vi "ReCalc V0.09.vi"() -> ()   [LabVIEW 2014]
uses:
  <vilib>/Utility/miscctls.llb/LVPointTypeDef.ctl
  <vilib>/Utility/NIReport.llb/Append Report Text (str wrap).vi
  <vilib>/Utility/xml.llb/Write to XML File(string).vi
  <vilib>/Utility/xml.llb/Read From XML File(string).vi
  <vilib>/Analysis/3filter.llb/IIR Filter (DBL).vi
  <vilib>/Utility/NIReport.llb/NI_report.lvclass
  <vilib>/Analysis/NI_AALBase.lvlib
  <vilib>/Analysis/NI_AALPro.lvlib
panel:
  in  "Speichern":bool
  out "aus Getriebe & Reifen":bool
  out "aus Zündsignal":bool=TRUE
  out "Reifenumfang [m]":dbl=1.222
  out "Getriebe [1:]":dbl=5.343
  out "Zündung [Imp/U]":u8=1
  out "Rolle [Inkr/U]":u16=200
  out "Luftdruck [mbar]":dbl=1013.0
  out "Luftfeuchtigkeit [%]":dbl=50.0
  out "Lufttemperatur [°C]":dbl=20.0
  in  "Berechnen":bool
  in  "Stopp":bool
  in  "Rollenträgheit [kgm²]":dbl=0.402
  in  "Polynom":u8=15
  in  "Gl. Mittelwert":u8=35
  in  "Differenzenquotient":u8=12
  in  "n vom Gas [1/min]":dbl=5000.0
  out "Rollenumfang [m]":dbl=0.613 format="%.3f"
  in  "nmax [1/min]":dbl=11000.0
  in  "nmin [1/min]":dbl=3000.0
  out "Datum, Zeit":string
  out "Untersetzung:":dbl=2.68 format="%.2f"
  in  "Drucken":bool
  out "Pmax":string
  out "Ergebnis":string
  out "Fahrzeugdaten":string
  out "XY-Graph":cluster{dbl[], dbl[]}[](graph)
  in  "Öffnen":bool
  out "korr":dbl
  out "[s]":dbl=5.0
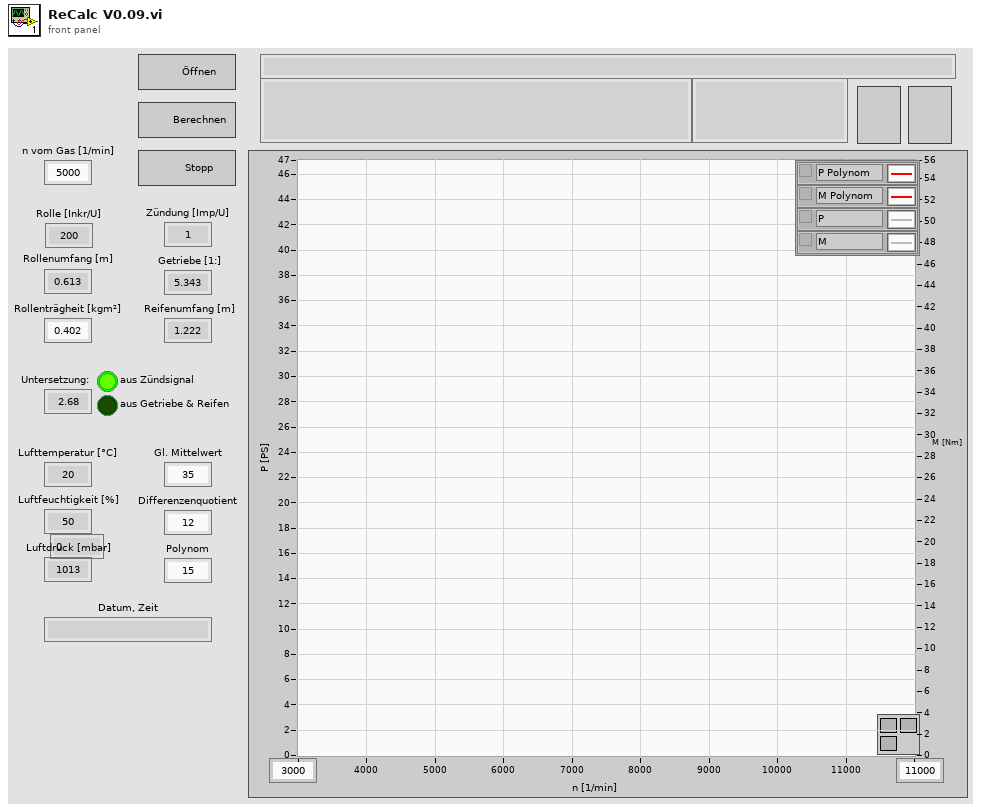
[diagram p1: front panel]
types:
  T1 = typedef "LVPointTypeDef.ctl" = cluster{"Horizontal":i16, "Vertical":i16}
  T2 = enum16{"Kleinste Quadrate", "Kleinestes absolutes Reiduum", "Biquadrat"}
  T3 = cluster{"Fahrzeugdaten":string, "Value":string, "Value":u16, "Value":dbl, "Value":dbl, "Value":u8, "Value":dbl, "Value":dbl, "Value":dbl, "Value":u8, "Value":u8, "Value":u8, dbl, dbl, "Value":dbl, "Value":dbl, "Value":dbl, dbl[], dbl[], "Best Polynomial Fit":dbl[], dbl[], "Value":bool, "Value":dbl, "Value":dbl, "Value":dbl, "Value":dbl, dbl[], i32[]}
  T4 = cluster{string, string, u16, dbl, dbl, u8, dbl, dbl, dbl, u8, u8, u8, dbl, dbl, dbl, dbl, dbl, dbl[], dbl[], dbl[], dbl[], bool, dbl, dbl, dbl, dbl, dbl[], i32[]}
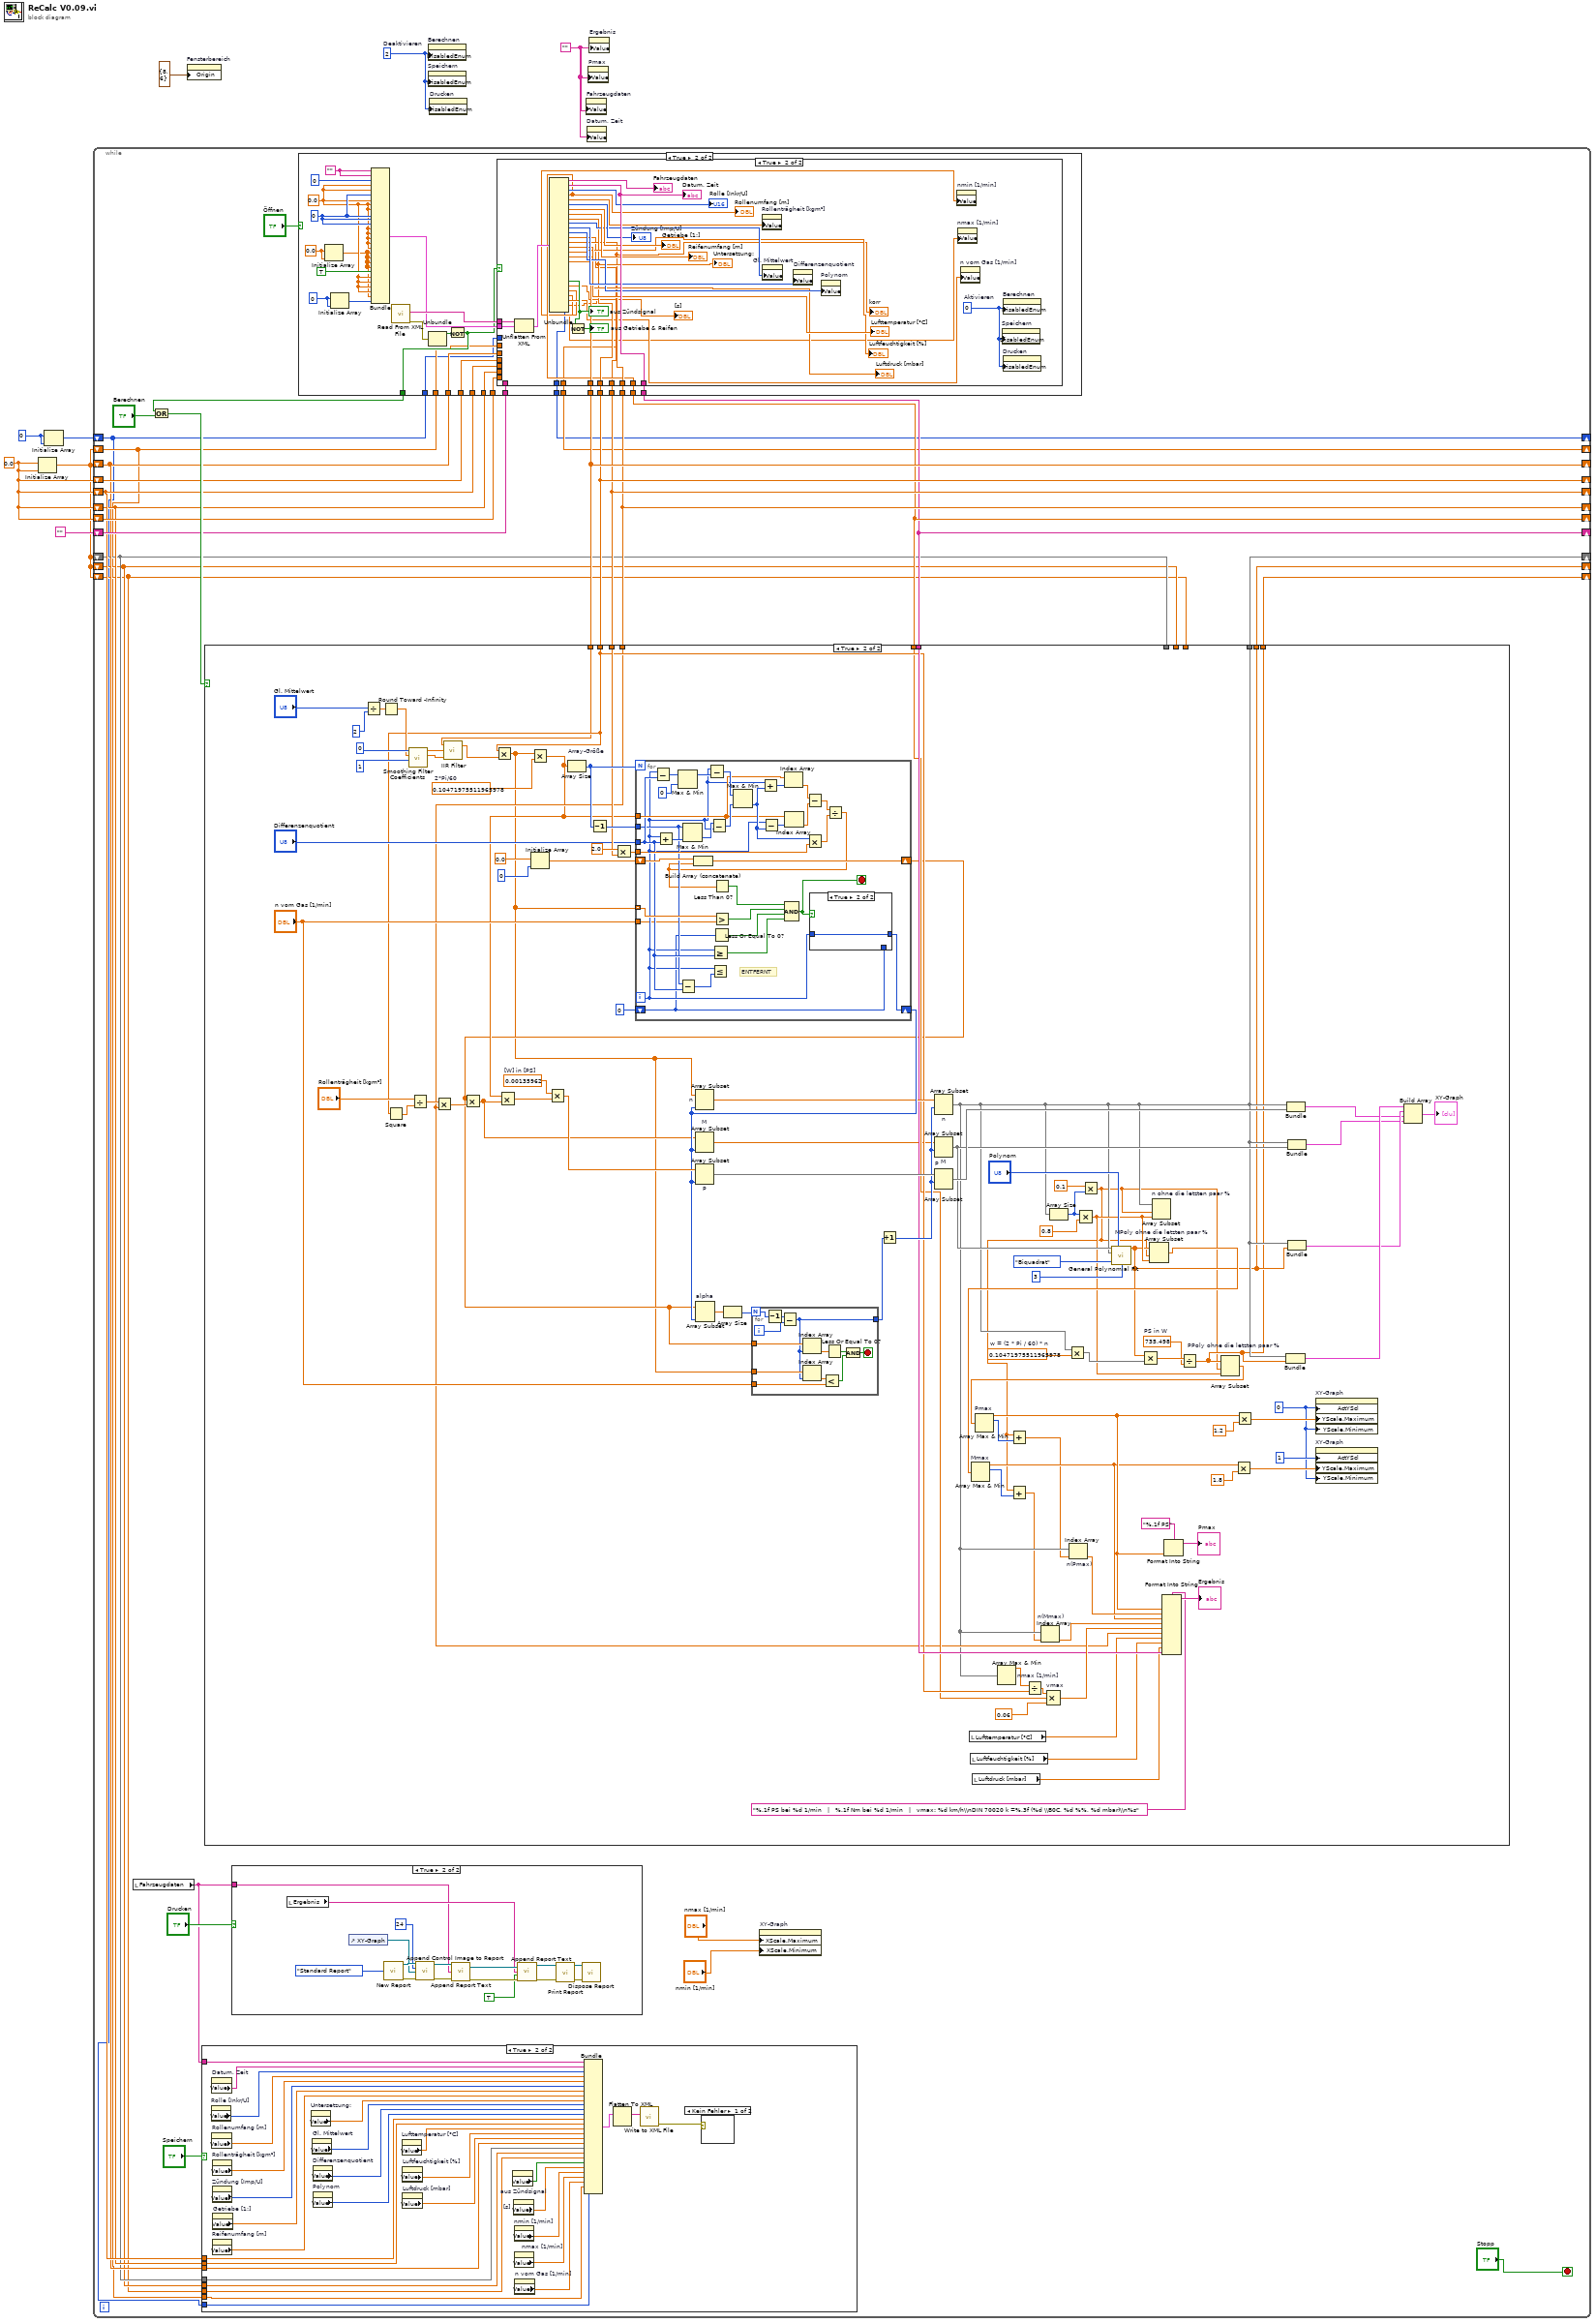
[diagram p0: block diagram]
diagram:
  w1 = 0
  w7 = 0.0
  w4 = 2  # Deaktivieren
  w8 = ""
  n1 = Initialize Array(w7, w7) -> (w3:dbl[])
  n2 = Initialize Array(w1, w1) -> (w2:i32[])
  n3 = while {
    shift-right: [w32] -> _
    shift-left: w3 -> [w21]
    shift-right: [w31] -> _
    shift-left: w7 -> [w35]
    shift-right: [w30] -> _
    shift-left: w7 -> [w23]
    shift-right: [w29] -> _
    shift-left: w7 -> [w22]
    shift-right: [w28] -> _
    shift-left: w7 -> [w34]
    shift-right: [w27] -> _
    shift-left: "" -> [w33]
    shift-right: [w18] -> _
    shift-left: w3 -> [w15]
    shift-right: [w17] -> _
    shift-left: w3 -> [w14]
    shift-right: [w16] -> _
    shift-left: w3 -> [w13]
    shift-right: [w12] -> _
    shift-left: w3 -> [w11]
    shift-right: [w10] -> _
    shift-left: w2 -> [w9]
    stop <- "Stopp" stop-if-true
    n4 = local read "Fahrzeugdaten"() -> (w24:string)
    n5 = case shown="True" "Speichern" {
      tunnel: w24 -> [_ w69]
      tunnel: w23 -> [_ w57]
      tunnel: w22 -> [_ w56]
      tunnel: w21 -> [_ w52]
      tunnel: w15 -> [_ w51]
      tunnel: w14 -> [_ w50]
      tunnel: w13 -> [_ w49]
      tunnel: w11 -> [_ w42]
      tunnel: w9 -> [_ w41]
      frame False {
      }
      frame True {
        n6 = property on="Rolle [Inkr/U]" class="DigWert (strikt)"() -> ("Value"=w67:u16)  [unwired: 2 in, 2 out]
        n7 = property on="Datum, Zeit" class="Str"() -> ("Value"=w68:string)  [unwired: 2 in, 2 out]
        n8 = property on="Rollenumfang [m]" class="DigWert (strikt)"() -> ("Value"=w66:dbl)  [unwired: 2 in, 2 out]
        n9 = property on="Rollenträgheit [kgm²]" class="DigWert (strikt)"() -> ("Value"=w65:dbl)  [unwired: 2 in, 2 out]
        n10 = property on="Zündung [Imp/U]" class="DigWert (strikt)"() -> ("Value"=w64:u8)  [unwired: 2 in, 2 out]
        n11 = property on="Reifenumfang [m]" class="DigWert (strikt)"() -> ("Value"=w62:dbl)  [unwired: 2 in, 2 out]
        n12 = property on="Getriebe [1:]" class="DigWert (strikt)"() -> ("Value"=w63:dbl)  [unwired: 2 in, 2 out]
        n13 = property on="Untersetzung:" class="DigWert (strikt)"() -> ("Value"=w61:dbl)  [unwired: 2 in, 2 out]
        n14 = property on="Gl. Mittelwert" class="DigWert (strikt)"() -> ("Value"=w60:u8)  [unwired: 2 in, 2 out]
        n15 = property on="Differenzenquotient" class="DigWert (strikt)"() -> ("Value"=w59:u8)  [unwired: 2 in, 2 out]
        n16 = property on="Polynom" class="DigWert (strikt)"() -> ("Value"=w58:u8)  [unwired: 2 in, 2 out]
        n17 = property on="Lufttemperatur [°C]" class="DigWert (strikt)"() -> ("Value"=w55:dbl)  [unwired: 2 in, 2 out]
        n18 = property on="Luftfeuchtigkeit [%]" class="DigWert (strikt)"() -> ("Value"=w54:dbl)  [unwired: 2 in, 2 out]
        n19 = property on="Luftdruck [mbar]" class="DigWert (strikt)"() -> ("Value"=w53:dbl)  [unwired: 2 in, 2 out]
        n20 = property on="aus Zündsignal" class="Bool. (strikt)"() -> ("Value"=w48:bool)  [unwired: 2 in, 2 out]
        n21 = property on="[s]" class="DigWert (strikt)"() -> ("Value"=w47:dbl)  [unwired: 2 in, 2 out]
        n22 = property on="nmin [1/min]" class="DigWert (strikt)"() -> ("Value"=w46:dbl)  [unwired: 2 in, 2 out]
        n23 = property on="nmax [1/min]" class="DigWert (strikt)"() -> ("Value"=w45:dbl)  [unwired: 2 in, 2 out]
        n24 = property on="n vom Gas [1/min]" class="DigWert (strikt)"() -> ("Value"=w44:dbl)  [unwired: 2 in, 2 out]
        n25 = Bundle("Fahrzeugdaten"=w69, "Value"=w68, "Value"=w67, "Value"=w66, "Value"=w65, "Value"=w64, "Value"=w63, "Value"=w62, "Value"=w61, "Value"=w60, "Value"=w59, "Value"=w58, w57, w56, "Value"=w55, "Value"=w54, "Value"=w53, w52, w51, "Best Polynomial Fit"=w50, w49, "Value"=w48, "Value"=w47, "Value"=w46, "Value"=w45, "Value"=w44, w42, w41) -> (w70:T3)  [unwired: 1 in]
        n26 = Flatten To XML(anything=w70) -> (xml string=w71:string)
        n27 = call-poly <vilib>:"Write to XML File.vi"("XML Input"=w71) -> ("error out"=w43:errorcluster)  [unwired: 8 in, 2 out]
        n28 = case shown="Kein Fehler" w43 {
          frame No Error {
          }
          frame Error {
          }
        }
      }
    }
    n29 = case shown="True" "Drucken" {
      tunnel: w24 -> [_ w74]
      frame False {
      }
      frame True {
        n30 = local read "Ergebnis"() -> (w75:string)
        n31 = control-ref of="XY-Graph"() -> (w78:refnum<vi>)
        n32 = call <vilib>:"New Report.vi"("report type"=enum16{"Standard Report", "HTML"}."Standard Report") -> ("report out"=w87:refnum<class "NI_report.lvclass">, "error out"=w86:errorcluster)  [unwired: 13 in]
        n33 = call-dynamic "Append Control Image to Report.vi"("report in"=w87, "image depth"=24, "ctrl reference"=w78, "error in (no error)"=w86) -> ("report out"=w82:refnum<class "NI_report.lvclass">, "error out"=w83:errorcluster)  [unwired: 8 in, 2 out]
        n34 = call-poly <vilib>:"Append Report Text.vi"("report in"=w82, "text"=w74, "error in (no error)"=w83) -> ("report out"=w81:refnum<class "NI_report.lvclass">, "error out"=w80:errorcluster)  [unwired: 9 in, 2 out]
        n35 = call-poly <vilib>:"Append Report Text.vi"("report in"=w81, "text"=w75, "append on new line? (F)"=TRUE, "error in (no error)"=w80) -> ("report out"=w73:refnum<class "NI_report.lvclass">, "error out"=w72:errorcluster)  [unwired: 8 in, 2 out]
        n36 = call-dynamic "Print Report.vi"("report in"=w73, "error in (no error)"=w72) -> ("report out"=w84:refnum<class "NI_report.lvclass">, "error out"=w85:errorcluster)  [unwired: 12 in]
        n37 = call-dynamic "Dispose Report.vi"("report in"=w84, "error in (no error)"=w85) -> ()  [unwired: 13 in, 1 out]
      }
    }
    n38 = case shown="True" "Öffnen" {
      selector: "Öffnen" -> [w239 _]
      tunnel: [w238 w259] -> w32
      tunnel: [w237 w258] -> w31
      tunnel: [w236 w255] -> w30
      tunnel: [w235 w257] -> w29
      tunnel: [w239 w253] -> w39
      tunnel: [w233 w263] -> w27
      tunnel: [w234 w256] -> w28
      tunnel: w21 -> [w238 w252]
      tunnel: w35 -> [w237 w251]
      tunnel: w23 -> [w236 w250]
      tunnel: w22 -> [w235 w248]
      tunnel: w34 -> [w234 w249]
      tunnel: w33 -> [w233 w247]
      tunnel: w11 -> [w232 w245]
      tunnel: [w232 w244] -> w12
      tunnel: [w231 w241] -> w10
      tunnel: w9 -> [w231 w240]
      frame False {
      }
      frame True {
        w242 = 0
        w261 = u8 0
        w266 = 0.0
        w254 = 0.0
        w267 = ""
        n39 = Initialize Array(w266, w266) -> (w246:dbl[])
        n40 = Initialize Array(w242, w242) -> (w243:i32[])
        n41 = Bundle(w267, w267, u16 0, w254, w254, w261, w254, w254, w254, w261, w261, w261, w254, w254, w254, w254, w254, w246, w246, w246, w246, TRUE, w254, w254, w254, w254, w246, w243) -> (w268:T4)  [unwired: 1 in]
        n42 = call-poly <vilib>:"Read From XML File.vi"() -> ("error out"=w265:errorcluster, "XML Elements"=w269:string)  [unwired: 9 in, 1 out]
        n43 = Unbundle(w265) -> ("status"=w264:bool)  [unwired: 2 out]
        n44 = Not(x=w264) -> (.not. x?=w253:bool)
        n45 = case shown="True" w253 {
          tunnel: w269 -> [_ w307]
          tunnel: w268 -> [_ w306]
          tunnel: [w272 w303] -> w263
          tunnel: [w277 w289] -> w259
          tunnel: [w276 w288] -> w258
          tunnel: [w273 w287] -> w257
          tunnel: [w274 w286] -> w256
          tunnel: [w275 w285] -> w255
          tunnel: w252 -> [w277 _]
          tunnel: w251 -> [w276 _]
          tunnel: w250 -> [w275 _]
          tunnel: w249 -> [w274 _]
          tunnel: w248 -> [w273 _]
          tunnel: w247 -> [w272 _]
          tunnel: w245 -> [w271 _]
          tunnel: [w271 w279] -> w244
          tunnel: [w270 w278] -> w241
          tunnel: w240 -> [w270 _]
          frame False {
          }
          frame True {
            w280 = 0  # Aktivieren
            n46 = Unflatten From XML(xml string=w307, type=w306) -> (value=w305:T4)  [unwired: 1 in, 1 out]
            n47 = Unbundle(w305) -> (→"Fahrzeugdaten":string, w303:string, →"Rolle [Inkr/U]":u16, w286:dbl, w298:dbl, →"Zündung [Imp/U]":u8, →"Getriebe [1:]":dbl, →"Reifenumfang [m]":dbl, w288:dbl, w295:u8, w294:u8, w293:u8, w285:dbl, w287:dbl, →"Lufttemperatur [°C]":dbl, →"Luftfeuchtigkeit [%]":dbl, →"Luftdruck [mbar]":dbl, w289:dbl[], w301:bool, →"[s]":dbl, w282:dbl, w281:dbl, w283:dbl, w279:dbl[], w278:i32[])  [unwired: 3 out]
            "Datum, Zeit" <- w303
            "Untersetzung:" <- w288
            "Rollenumfang [m]" <- w286
            "aus Zündsignal" <- w301
            "korr" <- w287
            n48 = Not(x=w301) -> (.not. x?=→"aus Getriebe & Reifen":bool)
            n49 = property on="Rollenträgheit [kgm²]" class="DigWert (strikt)"("Value"=w298) -> ()  [unwired: 2 in, 2 out]
            n50 = property on="Gl. Mittelwert" class="DigWert (strikt)"("Value"=w295) -> ()  [unwired: 2 in, 2 out]
            n51 = property on="Differenzenquotient" class="DigWert (strikt)"("Value"=w294) -> ()  [unwired: 2 in, 2 out]
            n52 = property on="Polynom" class="DigWert (strikt)"("Value"=w293) -> ()  [unwired: 2 in, 2 out]
            n53 = property on="nmin [1/min]" class="DigWert (strikt)"("Value"=w282) -> ()  [unwired: 2 in, 2 out]
            n54 = property on="nmax [1/min]" class="DigWert (strikt)"("Value"=w281) -> ()  [unwired: 2 in, 2 out]
            n55 = property on="n vom Gas [1/min]" class="DigWert (strikt)"("Value"=w283) -> ()  [unwired: 2 in, 2 out]
            n56 = property on="Speichern" class="Bool."("DisabledEnum"=w280) -> ()  [unwired: 2 in, 2 out]
            n57 = property on="Berechnen" class="Bool."("DisabledEnum"=w280) -> ()  [unwired: 2 in, 2 out]
            n58 = property on="Drucken" class="Bool."("DisabledEnum"=w280) -> ()  [unwired: 2 in, 2 out]
          }
        }
      }
    }
    n59 = Or(x=w39, y="Berechnen") -> (x .or. y?=w37:bool)
    n60 = case shown="True" w37 {
      tunnel: w32 -> [_ w120]
      tunnel: w30 -> [_ w163]
      tunnel: w27 -> [_ w128]
      tunnel: w31 -> [_ w127]
      tunnel: w28 -> [_ w126]
      tunnel: w29 -> [_ w125]
      tunnel: [w90 w99] -> w18
      tunnel: [w89 w98] -> w17
      tunnel: [w88 w97] -> w16
      tunnel: w15 -> [w90 _]
      tunnel: w14 -> [w89 _]
      tunnel: w13 -> [w88 _]
      frame False {
      }
      frame True {
        w137 = 0
        w147 = 735.498  # PS in W
        w152 = 0.10471975511965978  # w = (2 * Pi / 60) * n
        w168 = 0.00135962  # [W] in [PS]
        w177 = 0.10471975511965978  # 2*Pi/60
        n61 = Divide(x="Gl. Mittelwert", y=2) -> (x/y=w182:dbl)
        n62 = Round Toward -Infinity(1:w182) -> (0:w181:dbl)
        n63 = Square(x=w127) -> (x^2=w169:dbl)
        n64 = call <vilib>:"Smoothing Filter Coefficients.vi"("shape"=1, "half-width"=w181, "type"=0) -> ("forward coefficients"=w178:dbl[], "reverse coefficients"=w179:dbl[])  [unwired: 6 in, 1 out]
        n65 = Divide(x="Rollenträgheit [kgm²]", y=w169) -> (x/y=w166:dbl)
        n66 = Multiply(x=w166, y=w125) -> (x*y=w165:dbl)
        n67 = call-poly <vilib>:"IIR Filter.vi"("Forward Coefficients"=w178, "Reverse Coefficients"=w179, "X"=w120) -> ("Filtered X"=w119:dbl[])  [unwired: 1 in, 1 out]
        n68 = Multiply(x=w127, y=w119) -> (x*y=w91:dbl[])
        n69 = Multiply(x=w91, y=w177) -> (x*y=w118:dbl[])
        n70 = Initialize Array(0.0 ("y"), 0) -> (w170:dbl[])
        n71 = Array Size "Array-Größe"(array=w118) -> (size(s)=w175:i32)
        n72 = Decrement(x=w175) -> (x-1=w176:i32)
        n73 = Multiply(x=2.0, y=w163) -> (x*y=w174:dbl)
        n74 = for {
          N: w175 -> [_]
          tunnel: "Differenzenquotient" -> [w207]
          tunnel: w118 -> [w214]
          tunnel: w176 -> [w206]
          tunnel: w174 -> [w215]
          shift-right: [w211] -> w117
          shift-left: w170 -> [w212]
          tunnel: w91 -> [w209] mode=indexing
          tunnel: "n vom Gas [1/min]" -> [w198]
          shift-right: [w197] -> w157
          shift-left: 0 -> [w200]
          i -> [w201]
          stop <- w199 stop-if-true
          # "ENTFERNT"
          n75 = Subtract(x=w201, y=w207) -> (x-y=w228:i32)
          n76 = Add(x=w201, y=w207) -> (x+y=w222:i32)
          n77 = Max & Min(x=w228, y=0) -> (max(x,y)=w226:i32)  [unwired: 1 out]
          n78 = Subtract(x=w206, y=w207) -> (x-y=w208:i32)
          n79 = Max & Min(x=w206, y=w222) -> (min(x,y)=w223:i32)  [unwired: 1 out]
          n80 = Subtract(x=w201, y=w226) -> (x-y=w225:i32)
          n81 = Subtract(x=w223, y=w201) -> (x-y=w224:i32)
          n82 = Less Or Equal?(x=w201, y=w208) -> ()  [unwired: 1 out]
          n83 = Greater Or Equal?(x=w201, y=w207) -> (x >= y?=w204:bool)
          n84 = Less Or Equal To 0?(x=w200) -> (x <= 0?=w202:bool)
          n85 = Greater?(x=w209, y=w198) -> (0:w210:bool)
          n86 = Max & Min(x=w225, y=w224) -> (min(x,y)=w216:i32)  [unwired: 1 out]
          n87 = Add(x=w201, y=w216) -> (x+y=w221:i32)
          n88 = Subtract(x=w201, y=w216) -> (x-y=w220:i32)
          n89 = Index Array(array=w214, index=w221) -> (element=w218:dbl)
          n90 = Index Array(array=w214, index=w220) -> (element=w219:dbl)
          n91 = Subtract(x=w218, y=w219) -> (x-y=w217:dbl)
          n92 = Multiply(x=w216, y=w215) -> (x*y=w213:dbl)
          n93 = Divide(x=w217, y=w213) -> (x/y=w205:dbl)
          n94 = Build Array (concatenate)(w212, w205) -> (w211:dbl[])
          n95 = Less Than 0?(x=w205) -> (x < 0?=w203:bool)
          n96 = Compound Arithmetic op=AND(w203, w210, w202, w204) -> (w199:bool)
          n97 = case shown="True" w199 {
            tunnel: w201 -> [_ w230]
            tunnel: [w229 w230] -> w197
            tunnel: w200 -> [w229 _]
            frame False {
            }
            frame True {
            }
          }
        }
        n98 = Multiply(x=w117, y=w165) -> (x*y=w115:dbl[])
        n99 = Multiply(x=w118, y=w115) -> (x*y=w167:dbl[])
        n100 = Multiply(x=w168, y=w167) -> (x*y=w158:dbl[])
        n101 = Array Subset "n"(array=w91, length=w157) -> (w146:dbl[])  [unwired: 1 in]
        n102 = Array Subset "M"(array=w115, length=w157) -> (w116:dbl[])  [unwired: 1 in]
        n103 = Array Subset "P"(array=w158, length=w157) -> (w145:dbl[])  [unwired: 1 in]
        n104 = Array Subset "alpha"(array=w117, length=w157) -> (w159:dbl[])  [unwired: 1 in]
        n105 = Array Size(array=w159) -> (size(s)=w156:i32)
        n106 = for {
          N: w156 -> [w196]
          tunnel: w117 -> [w193]
          tunnel: w91 -> [w190]
          tunnel: "n vom Gas [1/min]" -> [w187]
          tunnel: [w185] -> w154
          i -> [w191]
          stop <- w186 stop-if-true
          n107 = Decrement(x=w196) -> (x-1=w195:i32)
          n108 = Subtract(x=w195, y=w191) -> (x-y=w185:i32)
          n109 = Index Array(array=w193, index=w185) -> (element=w194:dbl)
          n110 = Index Array(array=w190, index=w185) -> (element=w189:dbl)
          n111 = Less?(x=w189, y=w187) -> (x < y?=w188:bool)
          n112 = Less Or Equal To 0?(x=w194) -> (x <= 0?=w192:bool)
          n113 = And(x=w192, y=w188) -> (x .and. y?=w186:bool)
        }
        n114 = Increment(x=w154) -> (x+1=w144:i32)
        n115 = Array Subset "n"(array=w146, index=w144) -> (w99:dbl[])  [unwired: 1 in]
        n116 = Array Subset "M"(array=w116, index=w144) -> (w151:dbl[])  [unwired: 1 in]
        n117 = Array Subset "P"(array=w145, index=w144) -> (w153:dbl[])  [unwired: 1 in]
        n118 = local read "Lufttemperatur [°C]"() -> (w108:dbl)
        n119 = local read "Luftfeuchtigkeit [%]"() -> (w106:dbl)
        n120 = local read "Luftdruck [mbar]"() -> (w107:dbl)
        n121 = Array Max & Min "nmax [1/min]"(array=w99) -> (max value=w135:dbl)  [unwired: 3 out]
        n122 = Divide(x=w135, y=w127) -> (x/y=w134:dbl)
        n123 = Compound Arithmetic op=MULTIPLY "vmax"(w134, w126, 0.06) -> (w130:dbl)
        n124 = Array Size(array=w99) -> (size(s)=w101:i32)
        n125 = Multiply(x=w99, y=w152) -> (x*y=w136:dbl[])
        n126 = Multiply(x=w101, y=0.8) -> (x*y=w102:dbl)
        n127 = Multiply(x=0.1, y=w101) -> (x*y=w94:dbl)
        n128 = call <vilib>:"General Polynomial Fit.vi"("Y"=w151, "polynomial order"="Polynom", "X"=w99, "method"=T2."Biquadrat" ("Methode"), "algorithm"=3) -> ("Best Polynomial Fit"=w98:dbl[])  [unwired: 7 in, 3 out]
        n129 = Multiply(x=w98, y=w136) -> (x*y=w148:dbl[])
        n130 = Array Subset "MPoly ohne die letzten paar %"(array=w98, index=w94, length=w102) -> (w103:dbl[])
        n131 = Array Max & Min "Mmax"(array=w103) -> (max value=w123:dbl, max index (indices)=w95:i32)  [unwired: 2 out]
        n132 = Add(x=w94, y=w95) -> (x+y=w93:dbl)
        n133 = Index Array "n(Mmax)"(array=w99, index=w93) -> (element=w131:dbl)
        n134 = Array Subset "n ohne die letzten paar %"(array=w99, index=w94, length=w102) -> ()  [unwired: 1 out]
        n135 = Divide(x=w148, y=w147) -> (x/y=w97:dbl[])
        n136 = Array Subset "PPoly ohne die letzten paar %"(array=w97, index=w94, length=w102) -> (w104:dbl[])
        n137 = Array Max & Min "Pmax"(array=w104) -> (max value=w124:dbl, max index (indices)=w96:i32)  [unwired: 2 out]
        n138 = Add(x=w94, y=w96) -> (x+y=w92:dbl)
        n139 = Index Array "n(Pmax)"(array=w99, index=w92) -> (element=w132:dbl)
        n140 = Format Into String(format string="%.1f PS bei %d 1/min   |   %.1f Nm bei %d 1/min   |   vmax: %d km/h\\nDIN 70020 k =%.3f (%d \\B0C, %d %%, %d mbar)\\n%s" ("Format-String"), w124, w132, w123, w131, w130, w125, w108, w106, w107, w128) -> (resulting string=→"Ergebnis":string)  [unwired: 2 in, 1 out]
        n141 = Format Into String(format string="%.1f PS" ("Format-String"), w124) -> (resulting string=→"Pmax":string)  [unwired: 2 in, 1 out]
        n142 = Multiply(x=w123, y=1.8) -> (x*y=w138:dbl)
        n143 = Multiply(x=w124, y=1.2) -> (x*y=w139:dbl)
        n144 = Bundle(w99, w97) -> (w113:cluster{dbl[], dbl[]})  [unwired: 1 in]
        n145 = Bundle(w99, w153) -> (w111:cluster{dbl[], dbl[]})  [unwired: 1 in]
        n146 = Bundle(w99, w151) -> (w110:cluster{dbl[], dbl[]})  [unwired: 1 in]
        n147 = Bundle(w99, "Best Polynomial Fit"=w98) -> (w112:cluster{dbl[], "Best Polynomial Fit":dbl[]})  [unwired: 1 in]
        n148 = property on="XY-Graph" class="XYGraph (strikt)"("ActYScl"=w137, "YScale.Maximum"=w139, "YScale.Minimum"=w137) -> ()  [unwired: 2 in, 2 out]
        n149 = property on="XY-Graph" class="XYGraph (strikt)"("ActYScl"=1, "YScale.Maximum"=w138, "YScale.Minimum"=w137) -> ()  [unwired: 2 in, 2 out]
        n150 = Build Array(w113, w112, w111, w110) -> (→"XY-Graph":cluster{dbl[], "Best Polynomial Fit":dbl[]}[])
      }
    }
    n151 = property on="XY-Graph" class="XYGraph (strikt)"("XScale.Maximum"="nmax [1/min]", "XScale.Minimum"="nmin [1/min]") -> ()  [unwired: 2 in, 2 out]
  }
  n152 = property on="Fensterbereich" class="Bereich"("Origin"=T1 {"Horizontal"=8, "Vertical"=6}) -> ()  [unwired: 2 in, 2 out]
  n153 = property on="Berechnen" class="Bool."("DisabledEnum"=w4) -> ()  [unwired: 2 in, 2 out]
  n154 = property on="Speichern" class="Bool."("DisabledEnum"=w4) -> ()  [unwired: 2 in, 2 out]
  n155 = property on="Drucken" class="Bool."("DisabledEnum"=w4) -> ()  [unwired: 2 in, 2 out]
  n156 = property on="Fahrzeugdaten" class="Str"("Value"=w8) -> ()  [unwired: 2 in, 2 out]
  n157 = property on="Datum, Zeit" class="Str"("Value"=w8) -> ()  [unwired: 2 in, 2 out]
  n158 = property on="Pmax" class="Str"("Value"=w8) -> ()  [unwired: 2 in, 2 out]
  n159 = property on="Ergebnis" class="Str"("Value"=w8) -> ()  [unwired: 2 in, 2 out]
